vi "簇的使用(上).vi"() -> ()   [LabVIEW 2018]
panel:
  out "元素 2":cluster{string, bool}
  out "元素":T1
  out "输出簇 2":T2
  out "输出簇":T2
  out "枚举":enum16{"女", "男"}(ring)
  out "姓名":string
  out "学号":string
  in  "簇":T2
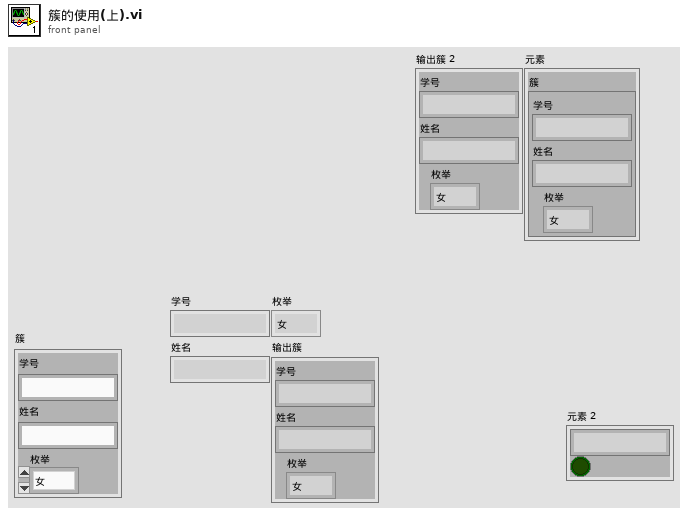
[diagram p1: front panel]
types:
  T1 = cluster{"簇":cluster{"学号":string, "姓名":string, "枚举":enum16{"女", "男"}}}
  T2 = cluster{"学号":string, "姓名":string, "枚举":enum16{"女", "男"}}
  T3 = cluster{"簇":cluster{"学号":string, "姓名":string, "枚举":enum16{"女", "男"}}}[]
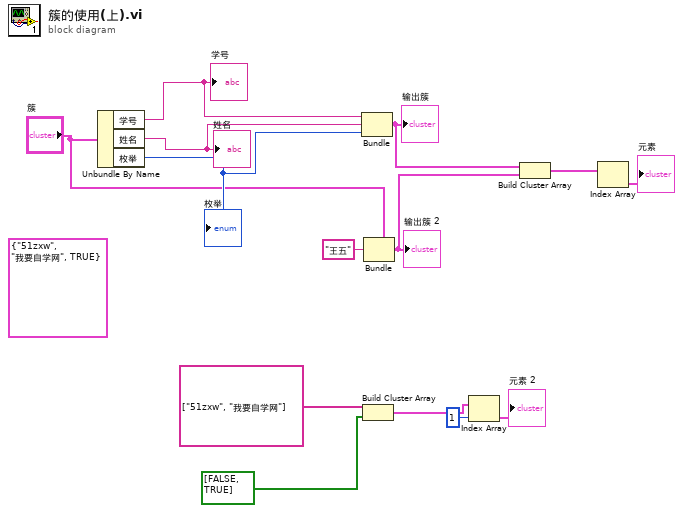
[diagram p0: block diagram]
diagram:
  (unwired) cluster{string, string, bool} {"51zxw", "我要自学网", TRUE}
  n1 = Unbundle By Name("簇") -> ("学号"=w14:string, "姓名"=w13:string, "枚举"=w12:enum16{"女", "男"})
  "学号" <- w14
  "姓名" <- w13
  "枚举" <- w12
  n2 = Bundle("学号"=w14, "姓名"=w13, "枚举"=w12) -> (w8:T2)  [unwired: 1 in]
  "输出簇" <- w8
  n3 = Build Cluster Array(string[] ["51zxw", "我要自学网"], bool[] [FALSE, TRUE]) -> (w3:cluster{string, bool}[])
  n4 = Bundle(cluster="簇", "姓名"="王五") -> (w9:T2)  [unwired: 2 in]
  "输出簇 2" <- w9
  n5 = Index Array(array=w3, index=1 ("索引")) -> (element=→"元素 2":cluster{string, bool})
  n6 = Build Cluster Array(w8, w9) -> (w7:T3)
  n7 = Index Array(array=w7) -> (element=→"元素":T1)  [unwired: 1 in]
